vi "StopLogging.vi"(8 "error in (no error)":errorcluster, 11 "DataLogger in":refnum<class "DataLogger.lvclass">) -> (0 "error out":errorcluster, 3 "DataLogger out":refnum<class "DataLogger.lvclass">)   [LabVIEW 2020, in "DataLogger.lvlib" / "DataLogger.lvclass"]
uses:
  DataLogger.lvclass
  C:/Program Files/National Instruments/LabVIEW 2020/vi.lib/ActorFramework/Actor/Actor.lvclass
  DataLogger.lvclass/DataLogger.ctl
  Hardware Abstraction Layer/Component/Device/Device/DataExchange.ctl
  <vilib>/ActorFramework/Actor/Actor.lvclass/Actor.ctl
  Interface/DataListener Messages/OnDataChange Msg/OnDataChange Msg.lvclass/OnDataChange Msg.ctl
  <vilib>/ActorFramework/Message Enqueuer/Message Enqueuer.lvclass/Message Enqueuer.ctl
  <vilib>/ActorFramework/Message Enqueuer/Enqueue.vi
  Interface/DataListener Messages/OnDataChange Msg/OnDataChange Msg.lvclass
  C:/Program Files/National Instruments/LabVIEW 2020/vi.lib/ActorFramework/Message/Message.lvclass
  <vilib>/ActorFramework/Message Priority Queue/Priority Enqueue.vi
  <vilib>/ActorFramework/Actor/Actor.lvclass
  Interface/DataListener/DataListener.lvclass
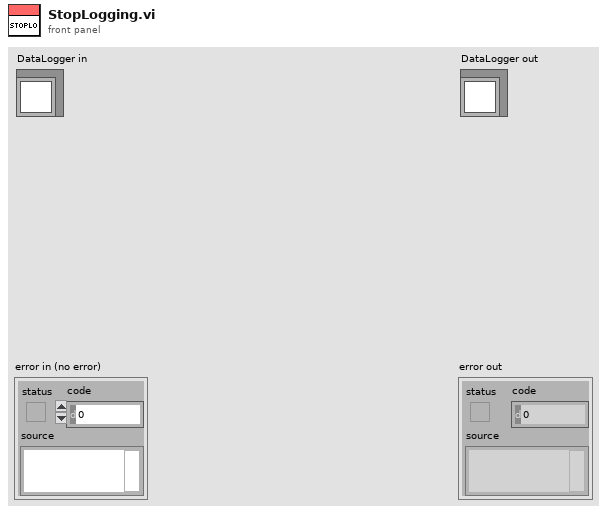
[diagram p1: front panel]
types:
  T1 = typedef "DataListener.lvclass/DataExchange.ctl" = cluster{"Source":string, "Destination":string, "Description":string, "value":variant}
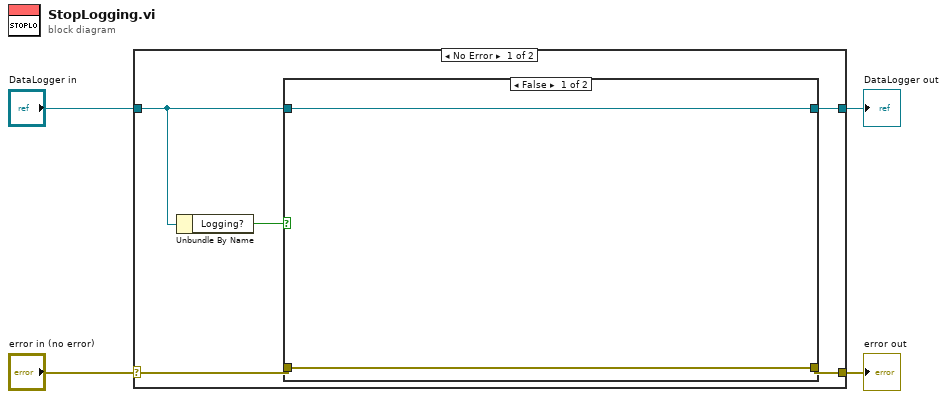
[diagram p0: block diagram]
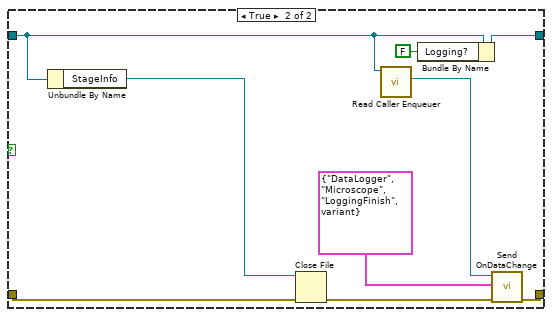
[diagram p2: hidden frame]
diagram:
  n1 = case shown="No Error" "error in (no error)" {
    selector: "error in (no error)" -> [w9 w22]
    tunnel: [w8 w22] -> w3
    tunnel: [w5 w21] -> w1
    tunnel: "DataLogger in" -> [w7 w21]
    frame No Error {
      n2 = Unbundle By Name(w7) -> ("Logging?"=w6:bool)
      n3 = case shown="False" w6 {
        tunnel: w9 -> [w10 w20]
        tunnel: [w10 w17] -> w8
        tunnel: w7 -> [w11 w14]
        tunnel: [w11 w13] -> w5
        frame False {
        }
        frame True {
          n4 = Unbundle By Name(w14) -> ("StageInfo"=w18:refnum<file>)
          n5 = Close File(refnum=w18, error in=w20) -> (error out=w19:errorcluster)  [unwired: 1 out]
          n6 = call <vilib>:"Read Caller Enqueuer.vi"("Actor"=w14) -> ("Caller Enqueuer"=w16:refnum<class "Message Enqueuer.lvclass">)  [unwired: 10 in]
          n7 = Bundle By Name(cluster=w14, "Logging?"=FALSE) -> (w13:refnum<class "DataLogger.lvclass">)
          n8 = call "Send OnDataChange.vi"("error in (no error)"=w19, "DataExchange"=T1 {"Source"="DataLogger", "Destination"="Microscope", "Description"="LoggingFinish", "value"=variant}, "Message Enqueuer"=w16) -> ("error out"=w17:errorcluster)  [unwired: 7 in, 1 out]
        }
      }
    }
    frame Error {
    }
  }
  "error out" <- w3
  "DataLogger out" <- w1
